vi "FlatToRichnixnet_grpc_ConvertFramesToSignalsSinglePointRequest.vi"(5 "OutputClusterType":T1, 11 "InputCluster":T4) -> (3 "OutputCluster":T1)   [LabVIEW 2025, in "grpc-xnet_client.lvlib"]
uses:
  nixnet_grpc_ConvertFramesToSignalsSinglePointRequest_Flat.ctl
  nidevice_grpc_Session_Flat.ctl
  nixnet_grpc_FrameBufferRequest_Flat.ctl
  nixnet_grpc_FrameRequest_Flat.ctl
  nixnet_grpc_FrameType.ctl
  nixnet_grpc_FrameFlags.ctl
  nixnet_grpc_EnetFrameRequest_Flat.ctl
  nixnet_grpc_EnetFrameType.ctl
  nixnet_grpc_EnetFlags.ctl
  nixnet_grpc_ConvertFramesToSignalsSinglePointRequest.ctl
  nidevice_grpc_Session.ctl
  nixnet_grpc_FrameBufferRequest.ctl
  nixnet_grpc_FrameBufferRequest_frame/nixnet_grpc_FrameBufferRequest_frame.lvclass
  grpc-xnet_client.lvlib
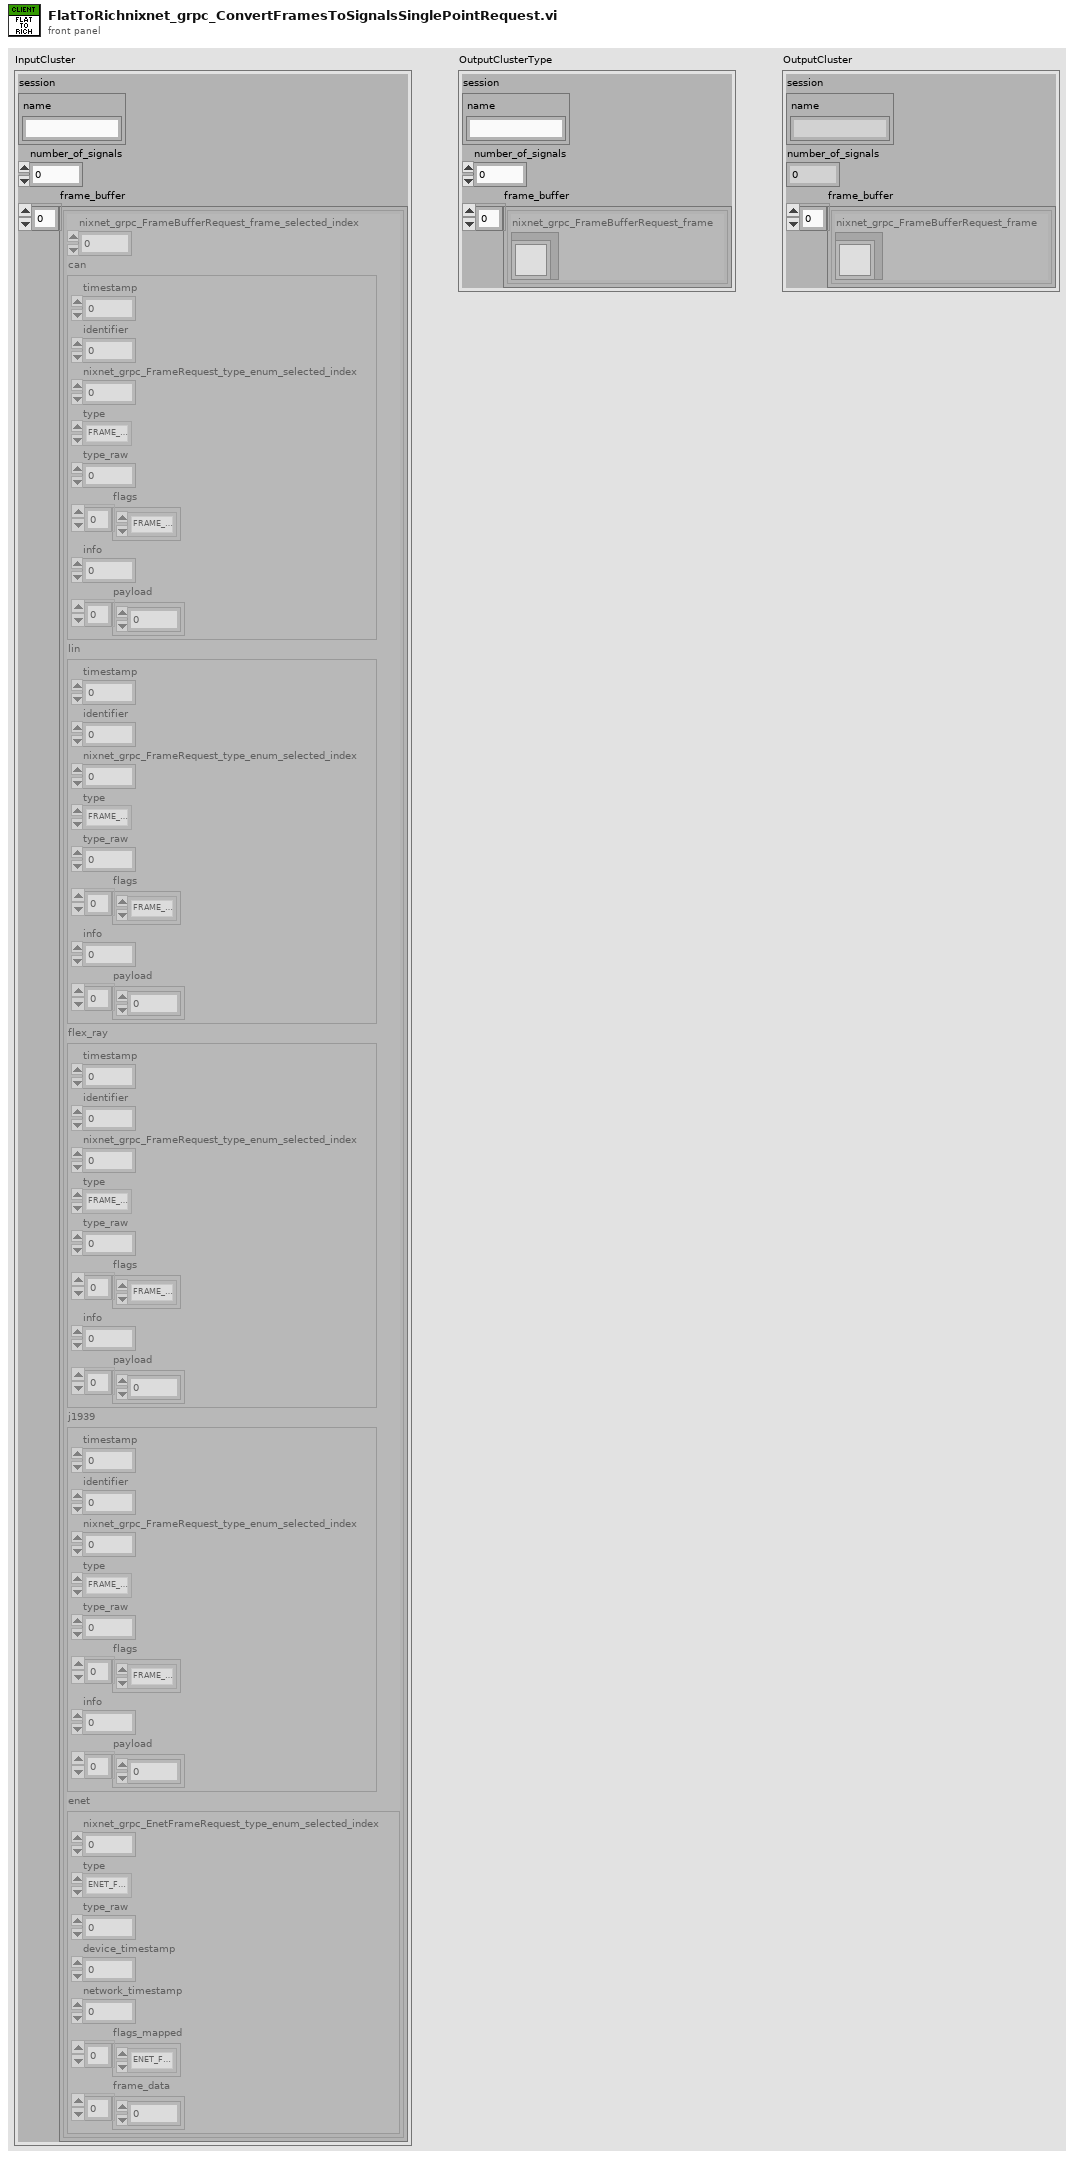
[diagram p1: front panel]
types:
  T1 = typedef "grpc-xnet_client.lvlib/nixnet_grpc_ConvertFramesToSignalsSinglePointRequest.ctl" = cluster{"session":T2, "number_of_signals":u32, "frame_buffer":T3[]}
  T2 = typedef "grpc-xnet_client.lvlib/nidevice_grpc_Session.ctl" = cluster{"name":string}
  T3 = typedef "grpc-xnet_client.lvlib/nixnet_grpc_FrameBufferRequest.ctl" = cluster{"nixnet_grpc_FrameBufferRequest_frame":refnum<class "nixnet_grpc_FrameBufferRequest_frame.lvclass">}
  T4 = typedef "grpc-xnet_client.lvlib/nixnet_grpc_ConvertFramesToSignalsSinglePointRequest_Flat.ctl" = cluster{"session":T5, "number_of_signals":u32, "frame_buffer":T6[]}
  T5 = typedef "grpc-xnet_client.lvlib/nidevice_grpc_Session_Flat.ctl" = cluster{"name":string}
  T6 = typedef "grpc-xnet_client.lvlib/nixnet_grpc_FrameBufferRequest_Flat.ctl" = cluster{"nixnet_grpc_FrameBufferRequest_frame_selected_index":i32, "can":T7, "lin":T7, "flex_ray":T7, "j1939":T7, "enet":T10}
  T7 = typedef "grpc-xnet_client.lvlib/nixnet_grpc_FrameRequest_Flat.ctl" = cluster{"timestamp":u64, "identifier":u32, "nixnet_grpc_FrameRequest_type_enum_selected_index":i32, "type":T8, "type_raw":u32, "flags":T9[], "info":u32, "payload":u8[]}
  T8 = typedef "grpc-xnet_client.lvlib/nixnet_grpc_FrameType.ctl" = enum32{"FRAME_TYPE_CAN_DATA", "FRAME_TYPE_CAN_REMOTE", "FRAME_TYPE_CAN_BUS_ERROR", "FRAME_TYPE_CAN20_DATA", "FRAME_TYPE_CANFD_DATA", "FRAME_TYPE_CANFDBRS_DATA", "FRAME_TYPE_FLEX_RAY_DATA", "FRAME_TYPE_FLEX_RAY_NULL", "FRAME_TYPE_FLEX_RAY_SYMBOL", "FRAME_TYPE_LIN_DATA", "FRAME_TYPE_LIN_BUS_ERROR", "FRAME_TYPE_LIN_NO_RESPONSE", "FRAME_TYPE_J1939_DATA", "FRAME_TYPE_SPECIAL_DELAY", "FRAME_TYPE_SPECIAL_LOG_TRIGGER", "FRAME_TYPE_SPECIAL_START_TRIGGER"}
  T9 = typedef "grpc-xnet_client.lvlib/nixnet_grpc_FrameFlags.ctl" = enum32{"FRAME_FLAGS_UNSPECIFIED", "FRAME_FLAGS_FLEX_RAY_STARTUP", "FRAME_FLAGS_FLEX_RAY_SYNC", "FRAME_FLAGS_FLEX_RAY_PREAMBLE", "FRAME_FLAGS_FLEX_RAY_CH_A", "FRAME_FLAGS_FLEX_RAY_CH_B", "FRAME_FLAGS_LIN_EVENT_SLOT", "FRAME_FLAGS_TRANSMIT_ECHO"}
  T10 = typedef "grpc-xnet_client.lvlib/nixnet_grpc_EnetFrameRequest_Flat.ctl" = cluster{"nixnet_grpc_EnetFrameRequest_type_enum_selected_index":i32, "type":T11, "type_raw":u32, "device_timestamp":u64, "network_timestamp":u64, "flags_mapped":T12[], "frame_data":u8[]}
  T11 = typedef "grpc-xnet_client.lvlib/nixnet_grpc_EnetFrameType.ctl" = enum32{"ENET_FRAME_TYPE_DATA", "ENET_FRAME_TYPE_DELAY", "ENET_FRAME_TYPE_FUTURE_TIME_WAIT"}
  T12 = typedef "grpc-xnet_client.lvlib/nixnet_grpc_EnetFlags.ctl" = enum32{"ENET_FLAGS_UNSPECIFIED", "ENET_FLAGS_TRANSMIT", "ENET_FLAGS_RECEIVE", "ENET_FLAGS_NETWORK_SYNCED", "ENET_FLAGS_ERROR"}
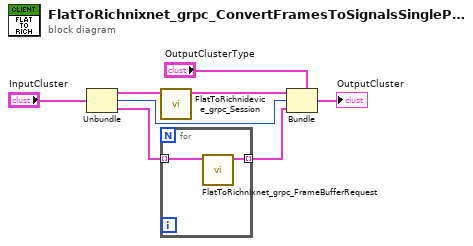
[diagram p0: block diagram]
diagram:
  n1 = Unbundle "Unbundle"("InputCluster") -> ("session"=w5:T5, "number_of_signals"=w3:u32, "frame_buffer"=w2:T6[])
  n2 = call "FlatToRichnidevice_grpc_Session.vi"("InputCluster"=w5) -> ("OutputCluster"=w4:T2)  [unwired: 10 in]
  n3 = for {
    tunnel: w2 -> [w10] mode=indexing
    tunnel: [w9] -> w1 mode=indexing
    n4 = call "FlatToRichnixnet_grpc_FrameBufferRequest.vi"("InputCluster"=w10) -> ("OutputCluster"=w9:T3)  [unwired: 10 in]
  }
  n5 = Bundle "Bundle"(cluster="OutputClusterType", "session"=w4, "number_of_signals"=w3, "frame_buffer"=w1) -> (→"OutputCluster":T1)
